vi "Get Terminal Counts.vi"(8 "error in (no error)":errorcluster, 11 "VI Refnum":refnum<vi>) -> (0 "error out":errorcluster, 3 "Terminal Counts":T1)   [LabVIEW 2026, in "VILab.lvlib"]
uses:
  VILab.lvlib
  CTLs/Terminal Counts.ctl
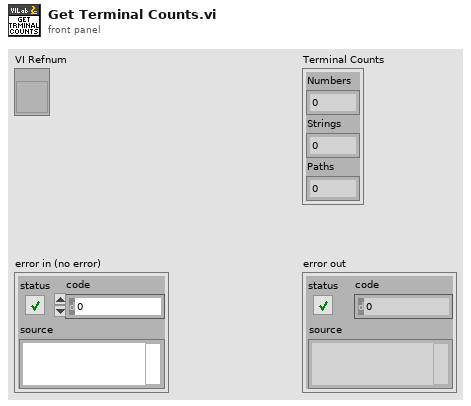
[diagram p1: front panel]
types:
  T1 = typedef "VILab.lvlib/Terminal Counts.ctl" = cluster{"Numbers":u32, "Strings":u32, "Paths":u32}
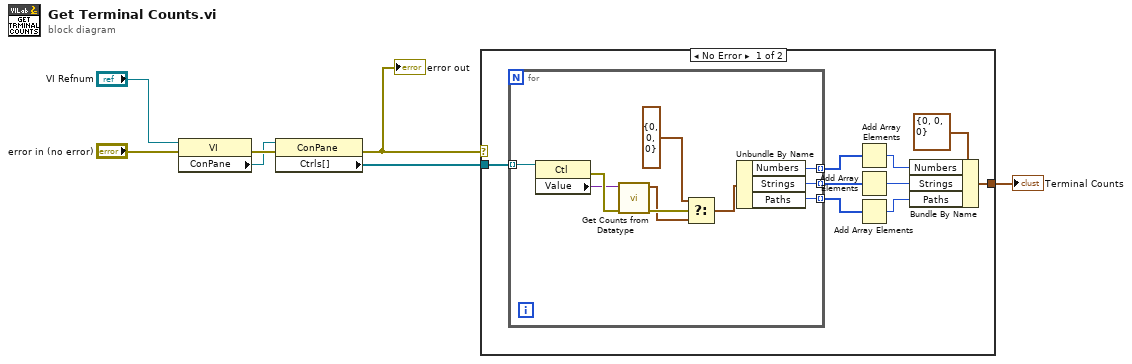
[diagram p0: block diagram]
diagram:
  n1 = property class="VI"(reference="VI Refnum", error in="error in (no error)") -> (error out=w6:errorcluster, "ConPane"=w3:refnum<vi>)  [unwired: 1 out]
  n2 = property class="ConPane"(reference=w3, error in=w6) -> (error out=w5:errorcluster, "Ctrls[]"=w2:refnum<vi>[])  [unwired: 1 out]
  "error out" <- w5
  n3 = case shown="No Error" w5 {
    tunnel: w2 -> [w16 _]
    tunnel: [w9 _] -> w1
    frame No Error {
      n4 = for {
        tunnel: w16 -> [w24] mode=indexing
        tunnel: [w22] -> w15 mode=indexing
        tunnel: [w21] -> w14 mode=indexing
        tunnel: [w20] -> w13 mode=indexing
        n5 = property class="Ctl"(reference=w24) -> (error out=w26:errorcluster, "Value"=w23:variant)  [unwired: 1 in, 1 out]
        n6 = call "Get Counts from Datatype.vi"("error in (no error)"=w26, "Type"=w23) -> ("error out"=w25:errorcluster, "Terminal Counts"=w19:T1)  [unwired: 8 in]
        n7 = Select(t=T1 {"Numbers"=0, "Strings"=0, "Paths"=0} ("Terminal Counts"), s=w25, f=w19) -> (s? t:f=w18:T1)
        n8 = Unbundle By Name(w18) -> ("Numbers"=w22:u32, "Strings"=w21:u32, "Paths"=w20:u32)
      }
      n9 = Add Array Elements(numeric array=w15) -> (sum=w12:u32)
      n10 = Add Array Elements(numeric array=w14) -> (sum=w11:u32)
      n11 = Add Array Elements(numeric array=w13) -> (sum=w10:u32)
      n12 = Bundle By Name(cluster=T1 {"Numbers"=0, "Strings"=0, "Paths"=0} ("Terminal Counts"), "Numbers"=w12, "Strings"=w11, "Paths"=w10) -> (w9:T1)
    }
    frame Error {
    }
  }
  "Terminal Counts" <- w1
